vi "Bit Encode LEDs.vi"(4 "E":bool, 6 "F":bool, 7 "G":bool, 8 "C":bool, 9 "D":bool, 10 "B":bool, 11 "A":bool) -> (3 "String":string)   [LabVIEW 2014, in "GEA2_Toolkit.lvlib"]
uses:
  Labview GEA2 Toolkit v2.1/library/GEA2_Toolkit.lvlib
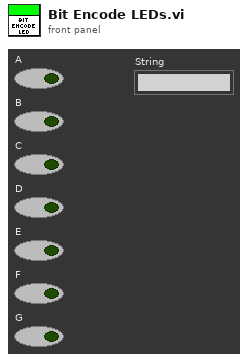
[diagram p1: front panel]
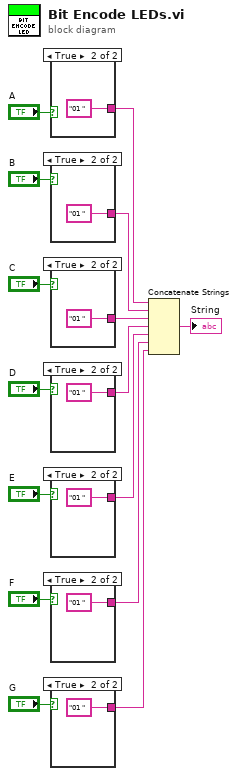
[diagram p0: block diagram]
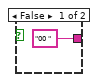
[diagram p2: hidden frame]
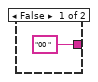
[diagram p3: hidden frame]
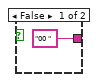
[diagram p4: hidden frame]
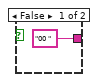
[diagram p5: hidden frame]
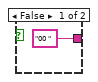
[diagram p6: hidden frame]
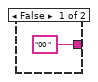
[diagram p7: hidden frame]
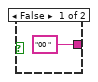
[diagram p8: hidden frame]
diagram:
  n1 = case shown="True" "A" {
    tunnel: ["00 " "01 "] -> w10
    frame False {
    }
    frame True {
    }
  }
  n2 = case shown="True" "B" {
    tunnel: ["00 " "01 "] -> w11
    frame False {
    }
    frame True {
    }
  }
  n3 = case shown="True" "C" {
    tunnel: ["00 " "01 "] -> w2
    frame False {
    }
    frame True {
    }
  }
  n4 = case shown="True" "D" {
    tunnel: ["00 " "01 "] -> w12
    frame False {
    }
    frame True {
    }
  }
  n5 = case shown="True" "E" {
    tunnel: ["00 " "01 "] -> w1
    frame False {
    }
    frame True {
    }
  }
  n6 = case shown="True" "F" {
    tunnel: ["00 " "01 "] -> w13
    frame False {
    }
    frame True {
    }
  }
  n7 = case shown="True" "G" {
    tunnel: ["00 " "01 "] -> w14
    frame False {
    }
    frame True {
    }
  }
  n8 = Concatenate Strings(w10, w11, w2, w12, w1, w13, w14) -> (→"String":string)
